vi "sv_Resample Filter Prototype (Continuous Swept-Sine).vi"(6 "alias free":bool, 7 "reset? (True)":bool=TRUE, 8 "error in (no error)":errorcluster, 9 "stop band attenuation [dB]":dbl=96.0, 10 "timing jitter":enum32{"Interpolation", "Rounding"}(ring)) -> (0 "error out":errorcluster, 2 "taps":i32, 3 "filter prototype":T1={"left wing"=[], "increment"=[], "max dec"=128, "timing jitter"=enum."Interpolation", "band limiting?"=TRUE} {"increment" format="%.2f"; "left wing" format="%.2f"})   [LabVIEW 2017, in "SoundVib_ContSweptSine.lvlib"]
doc: "Design a filter prototype for arbitrary resampling."
uses:
  <vilib>/addons/Sound and Vibration/svt_Continuous Swept Sine/SoundVib_ContSweptSine.lvlib
  <vilib>/addons/_NISVFA/_Shared subVIs/Controls/OAT Resample Filter Prototype.ctl
  <vilib>/addons/Sound and Vibration/Order Analysis/Resample Order Tracking/SoundVib_Resampling.lvlib
panel:
  in  "maximum decimation\nfactor (auto)":i32
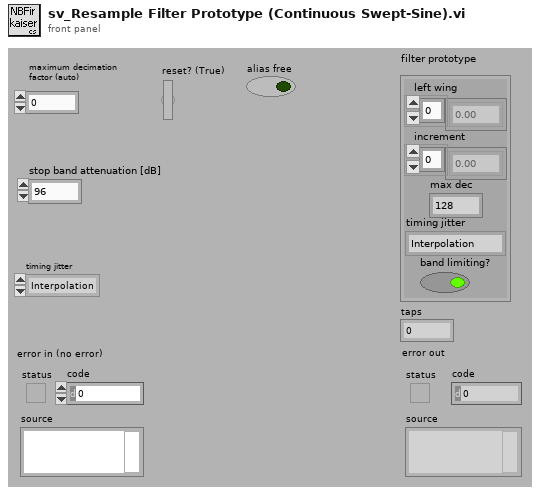
[diagram p1: front panel]
types:
  T1 = typedef "OAT Resample Filter Prototype.ctl" = cluster{"left wing":dbl[], "increment":dbl[], "max dec":i32, "timing jitter":enum32{"Interpolation", "Rounding"}, "band limiting?":bool}
  T2 = cluster{"maximum decimation\nfactor (auto)":i32, "alias free":bool, "stop band attenuation [dB]":dbl, "timing jitter":enum32{"Interpolation", "Rounding"}}
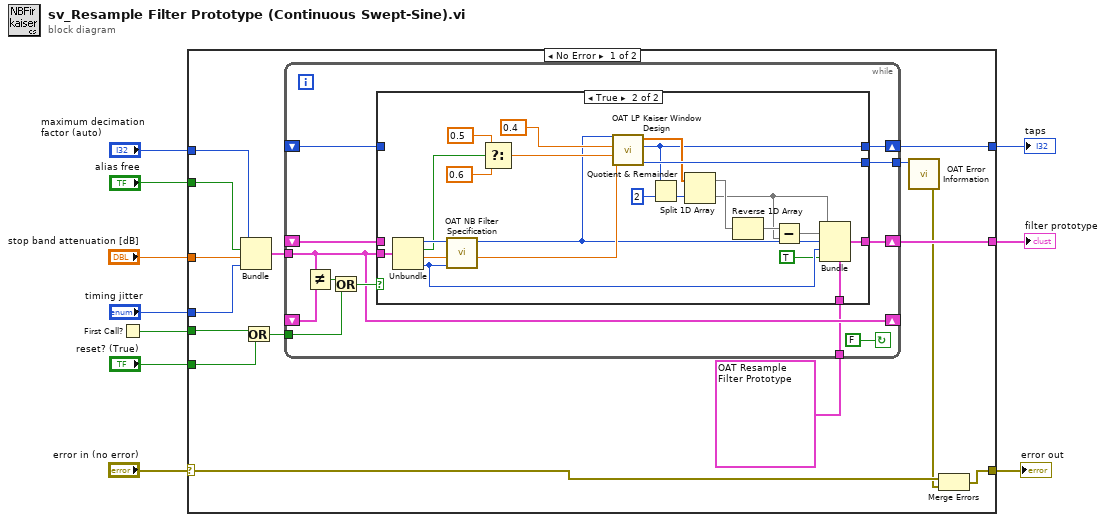
[diagram p0: block diagram]
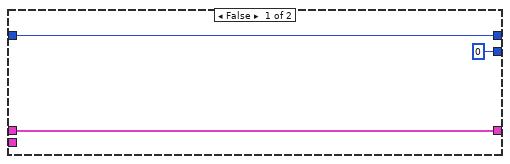
[diagram p2: hidden frame]
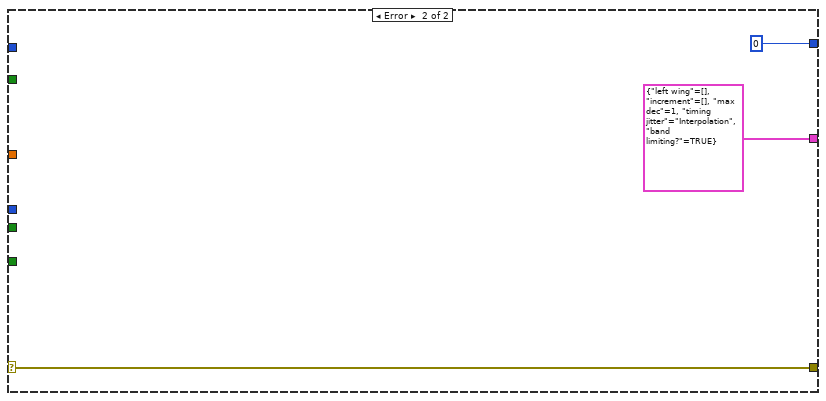
[diagram p3: hidden frame]
diagram:
  n1 = First Call?() -> (First Call?: T/F=w4:bool)
  n2 = case shown="No Error" "error in (no error)" {
    selector: "error in (no error)" -> [w14 w66]
    tunnel: [w25 T1 {"left wing"=[], "increment"=[], "max dec"=1, "timing jitter"=enum."Interpolation", "band limiting?"=TRUE} ("filter prototype")] -> w10
    tunnel: [w23 0 ("taps")] -> w9
    tunnel: "timing jitter" -> [w22 _]
    tunnel: "maximum decimation\nfactor (auto)" -> [w21 _]
    tunnel: "alias free" -> [w20 _]
    tunnel: "reset? (True)" -> [w17 _]
    tunnel: w4 -> [w16 _]
    tunnel: [w12 w66] -> w2
    tunnel: "stop band attenuation [dB]" -> [w11 _]
    frame No Error {
      n3 = Bundle("maximum decimation\nfactor (auto)"=w21, "alias free"=w20, "stop band attenuation [dB]"=w11, "timing jitter"=w22) -> (w24:T2)  [unwired: 1 in]
      n4 = Or(x=w16, y=w17) -> (x .or. y?=w15:bool)
      n5 = while {
        shift-right: [w37] -> w25
        shift-left: _ -> [w31]
        shift-right: [w28] -> _
        shift-left: _ -> [w29]
        tunnel: w24 -> [w28]
        shift-right: [w35] -> w23
        shift-left: _ -> [w30]
        tunnel: w15 -> [w34]
        tunnel: [w27] -> w19
        tunnel: T1 {"left wing"=array[915 elements], "increment"=array[914 elements], "max dec"=128, "timing jitter"=enum."Interpolation", "band limiting?"=TRUE} ("filter prototype") -> [w26]
        stop <- FALSE continue-if-true
        n6 = Not Equal?(x=w28, y=w29) -> (x != y?=w33:bool)
        n7 = Or(x=w33, y=w34) -> (x .or. y?=w32:bool)
        n8 = case shown="True" w32 {
          tunnel: [w40 w49] -> w35
          tunnel: [w39 w61] -> w37
          tunnel: w28 -> [_ w60]
          tunnel: w30 -> [w40 _]
          tunnel: w31 -> [w39 _]
          tunnel: [0 ("error") w52] -> w27
          tunnel: w26 -> [_ w45]
          frame False {
          }
          frame True {
            n9 = Unbundle(w60) -> ("maximum decimation\nfactor (auto)"=w57:i32, "alias free"=w54:bool, "stop band attenuation [dB]"=w56:dbl, "timing jitter"=w44:enum32{"Interpolation", "Rounding"})
            n10 = call <vilib>:"OAT NB Filter Specification.vi"("timing jitter"=w44, "stop band attenuation"=w56, "maximum decimation factor"=w57) -> ("A stop [dB]"=w55:dbl, "decimation factor"=w53:i32)  [unwired: 7 in]
            n11 = Select(t=0.5, s=w54, f=0.6) -> (s? t:f=w58:dbl)
            n12 = call <vilib>:"OAT LP Kaiser Window Design.vi"("A stop [dB]"=w55, "stopband"=w58, "passband"=0.4 ("low cutoff freq: fl"), "fs"=w53) -> ("error"=w52:i32, "taps"=w49:i32, "filter coefficients"=w51:dbl[])  [unwired: 5 in]
            n13 = Quotient & Remainder(x=w49, y=2) -> (floor(x/y)=w50:i32)  [unwired: 1 out]
            n14 = Split 1D Array(array=w51, index=w50) -> (first subarray=w47:dbl[], second subarray=w41:dbl[])
            n15 = Reverse 1D Array(array=w47) -> (reversed array=w42:dbl[])
            n16 = Subtract(x=w42, y=w41) -> (x-y=w46:dbl[])
            n17 = Bundle(cluster=w45, "left wing"=w41, "increment"=w46, "max dec"=w53, "timing jitter"=w44, "band limiting?"=TRUE) -> (w61:T1)
          }
        }
      }
      n18 = call <vilib>:"OAT Error Information.vi"("error code"=w19) -> ("error out"=w13:errorcluster)  [unwired: 6 in]
      n19 = Merge Errors(w14, w13) -> (w12:errorcluster)
    }
    frame Error {
    }
  }
  "filter prototype" <- w10
  "taps" <- w9
  "error out" <- w2
